vi "Cluster_Analysis.vi"(2 "Shift In":T1[](array[typedef])) -> (0 "Shift Out":T1[](array[typedef]))   [LabVIEW 2016]
uses:
  Controls/Shift_Cluster.ctl
  Controls/Inst_type.ctl
  Controls/XY_Plot_Cluster.ctl
  Globals/Meas_global.vi
  Globals/LDA_meas_global_1.vi
  Globals/LDA_meas_global_2.vi
  <vilib>/Analysis/NI_AALBase.lvlib
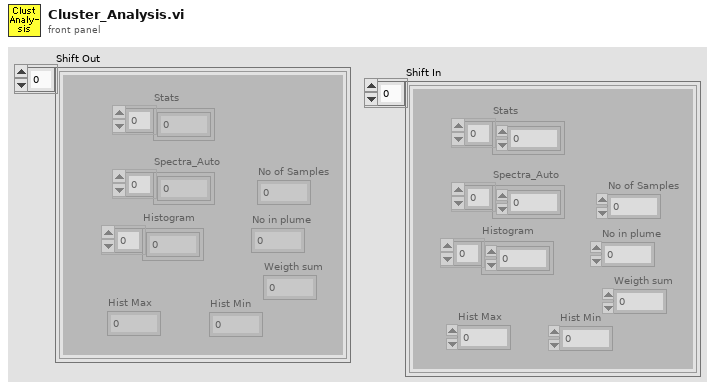
[diagram p1: front panel]
types:
  T1 = typedef "Shift_Cluster.ctl" = cluster{"Stats":dbl[], "Spectra_Auto":dbl[], "Histogram":dbl[], "Hist Max":dbl, "Hist Min":dbl, "No of Samples":i32, "No in plume":i32, "Weigth sum":dbl}
  T2 = typedef "Analysis_info_cluster.ctl" = cluster{"Colour":u32, "Inst type":T3, "Inst name":string, "Symbol":string, "Code name":string, "Extra Info":string, "Inst Array":T4, "Extra Titles":string[], "Extra Values":string[], "U":dbl, "u^2":dbl, "u^3":dbl, "u^4":dbl, "Skew_u":dbl, "Kurt_u":dbl, "Sd Error in Mean":dbl, "% u'/U":dbl, "X":dbl, "Y":dbl, "Z":dbl, "Timescale integral Estimate":dbl, "Sd Error in Variance":dbl, "Calib File":path, "Calib Constants":dbl[], "Output Position":bool, "Full Stats":bool, "Av Sampling Rate":dbl, "Av No of Samples":dbl, "Total Meas Time (s)":dbl, "ADAM Ch Name":string, "Max value":dbl, "Min value":dbl}
  T3 = typedef "Inst_type.ctl" = enum16{"Propeller anemometer", "Raw voltage", "Pressure Transducer", "Pitot-static tube", "Preston tube", "Hot wire", "Cross wire 1", "Cross wire 2", "Generic Linear", "Generic Polynomial", "Generic BackPoly", "Fast FID", "Thermocouple", "Cold wire", "Pulsed Wire", "LDA Vel", "LDA Tran time", "LDA Arr time", "Microphone"}
  T4 = typedef "Instrument_Array.ctl" = enum16{"PWA", "LDA", "Analogue"}
  T5 = typedef "Time_Trace_Cluster.ctl" = cluster{"Weighting":dbl[], "Time (s)":dbl[], "Voltage":dbl[], "Eng Values":dbl[]}
  T6 = typedef "XY_Plot_Cluster.ctl" = cluster{"First Name":string, "Second Name":string, "X axis name":string, "Y axis name":string, "X array":dbl[], "Y array":dbl[]}
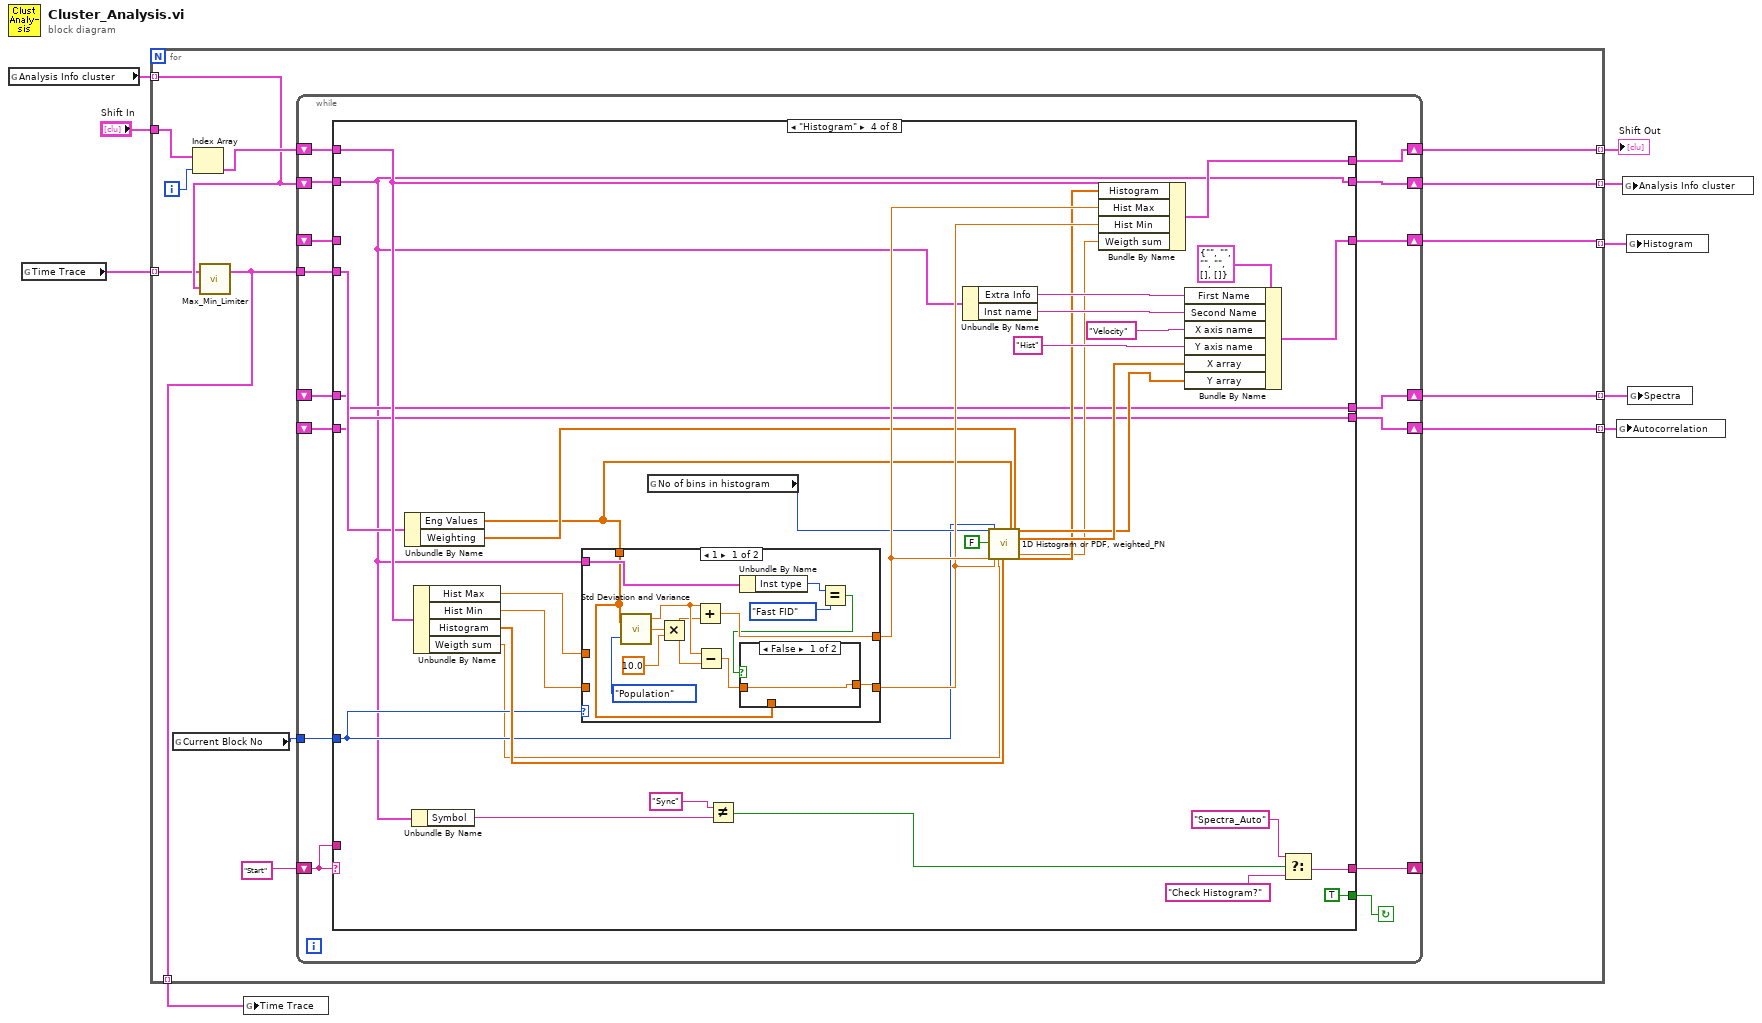
[diagram p0: block diagram]
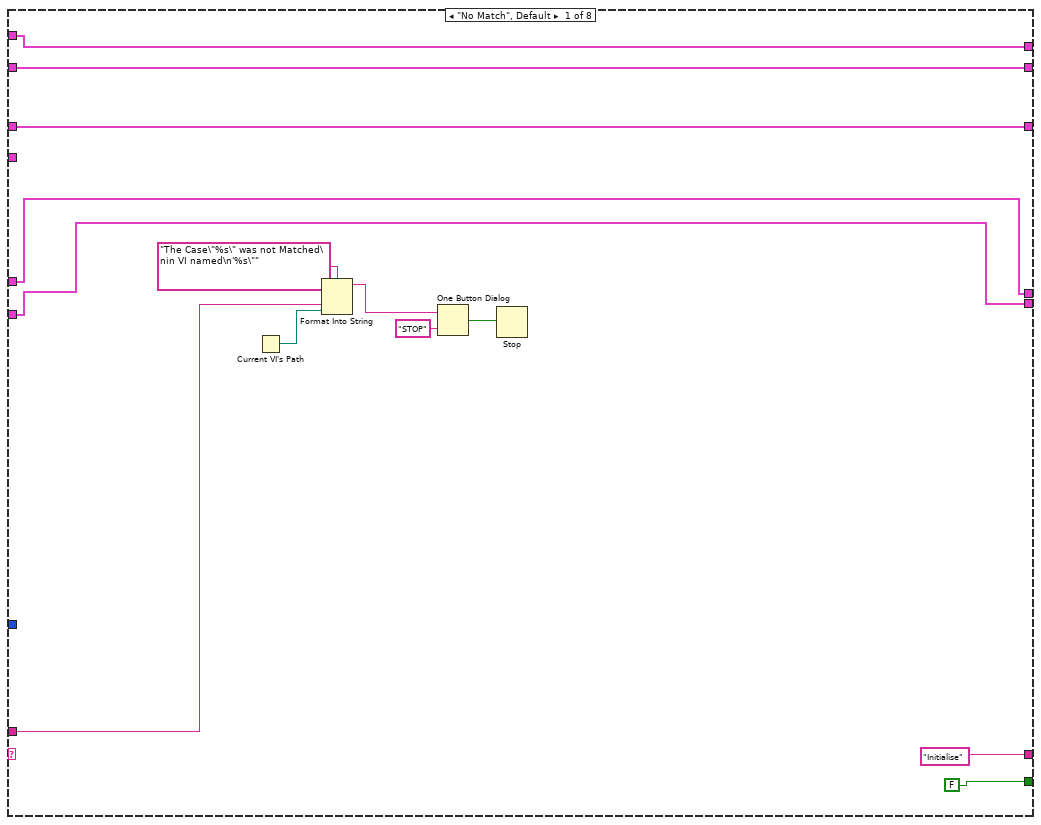
[diagram p2: hidden frame]
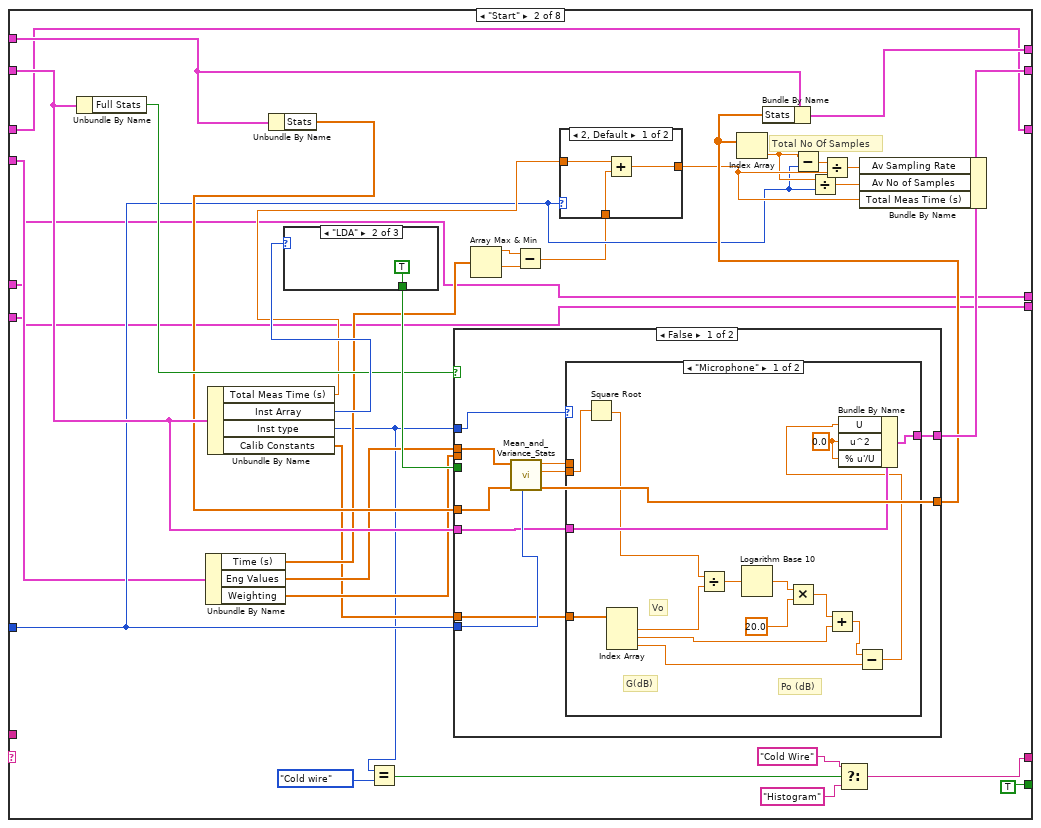
[diagram p3: hidden frame]
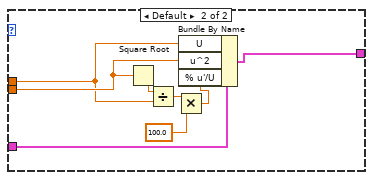
[diagram p5: hidden frame]
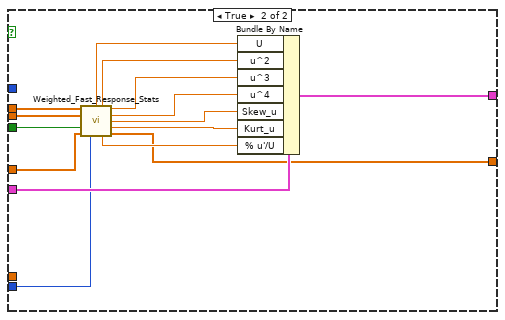
[diagram p6: hidden frame]
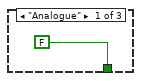
[diagram p7: hidden frame]
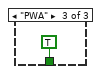
[diagram p8: hidden frame]
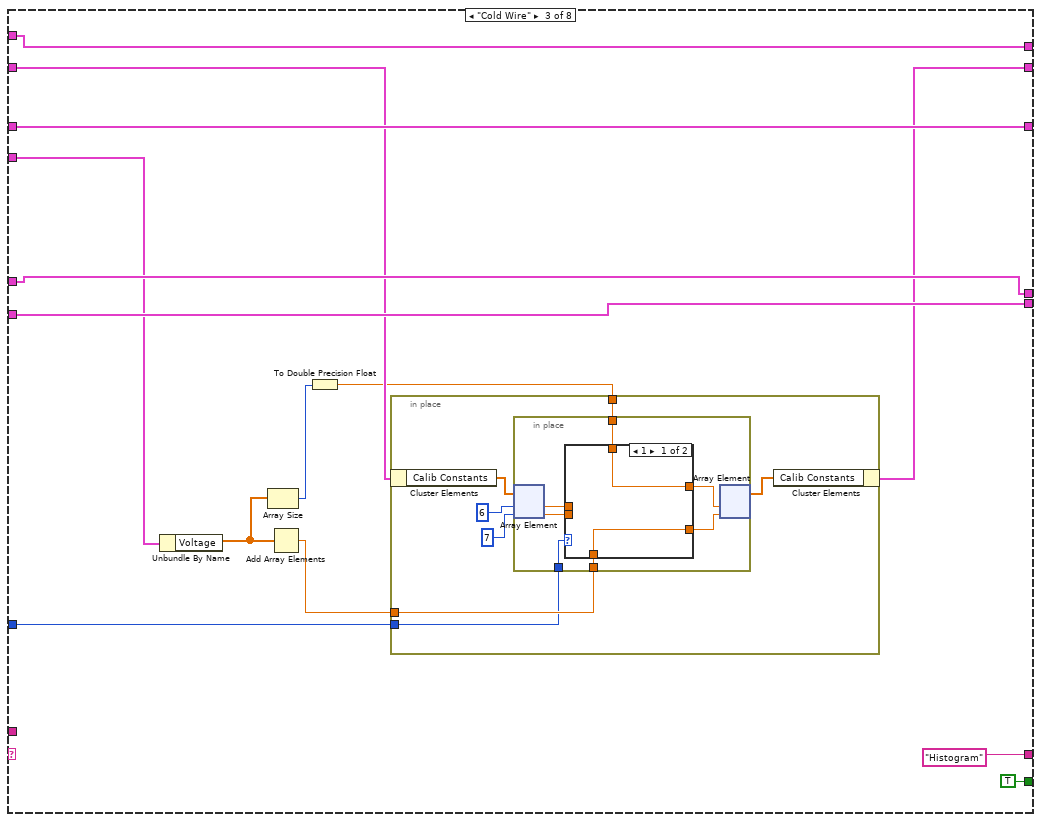
[diagram p9: hidden frame]
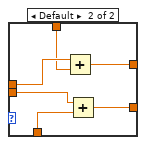
[diagram p10: hidden frame]
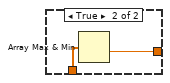
[diagram p11: hidden frame]
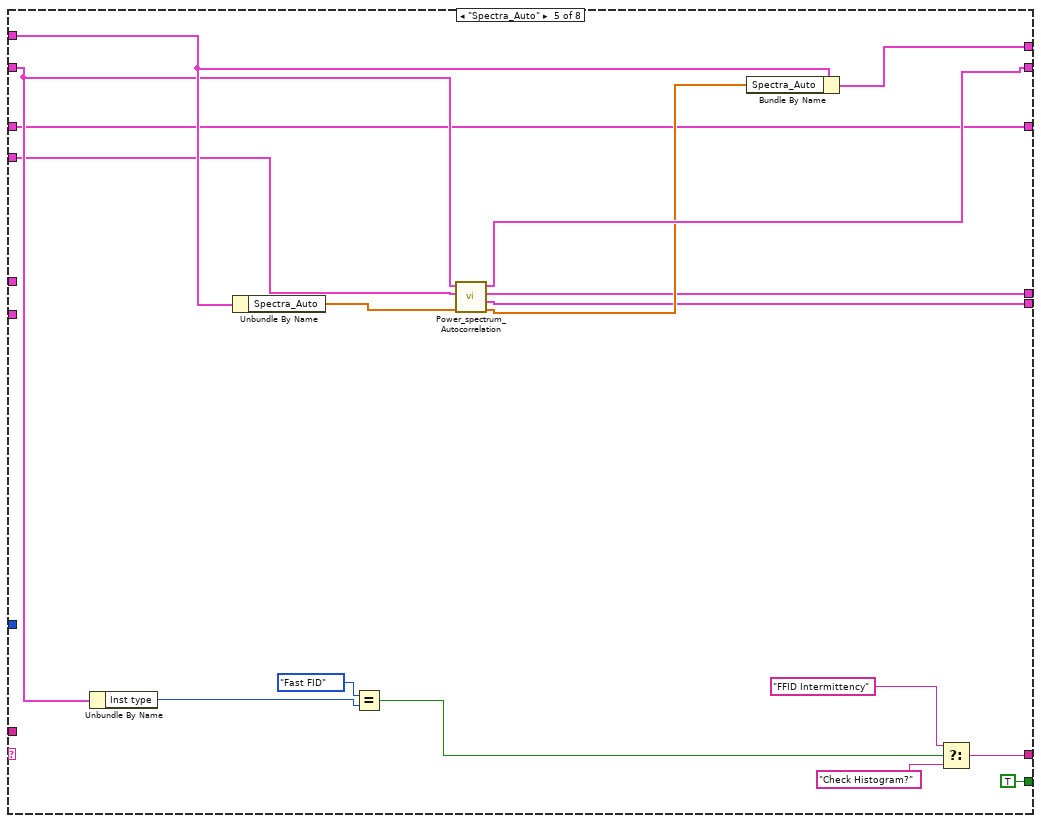
[diagram p13: hidden frame]
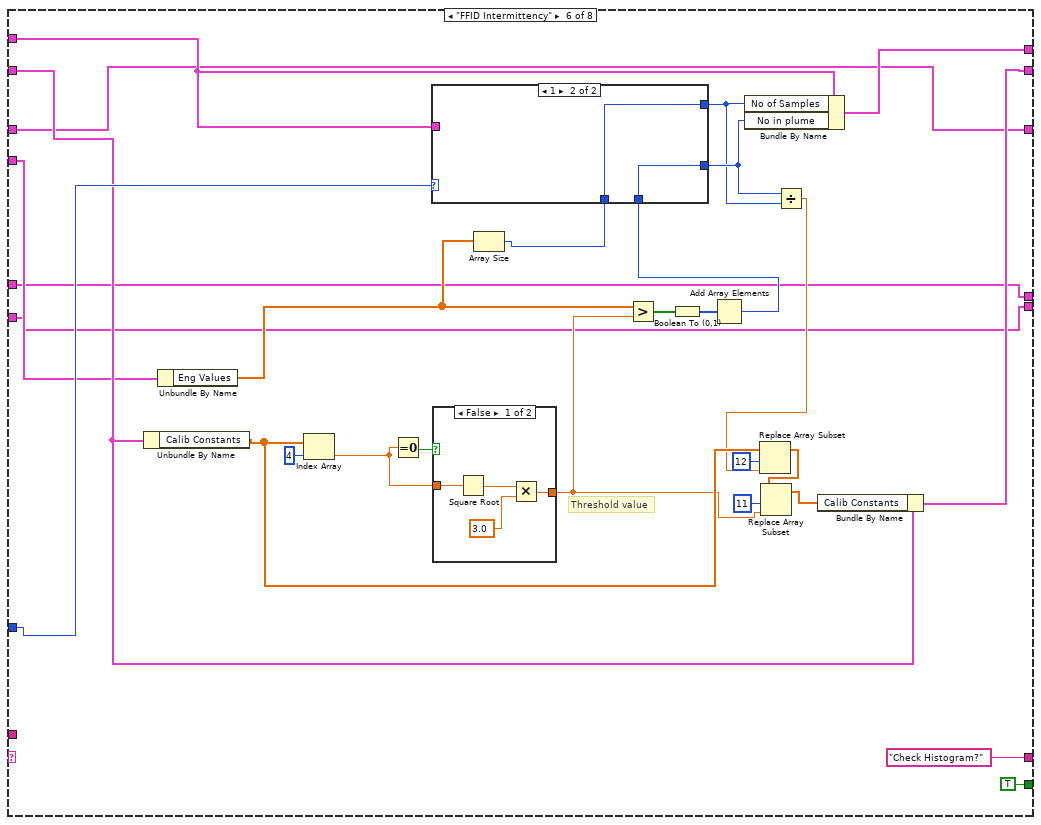
[diagram p14: hidden frame]
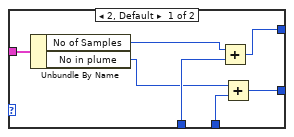
[diagram p15: hidden frame]
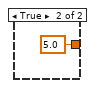
[diagram p16: hidden frame]
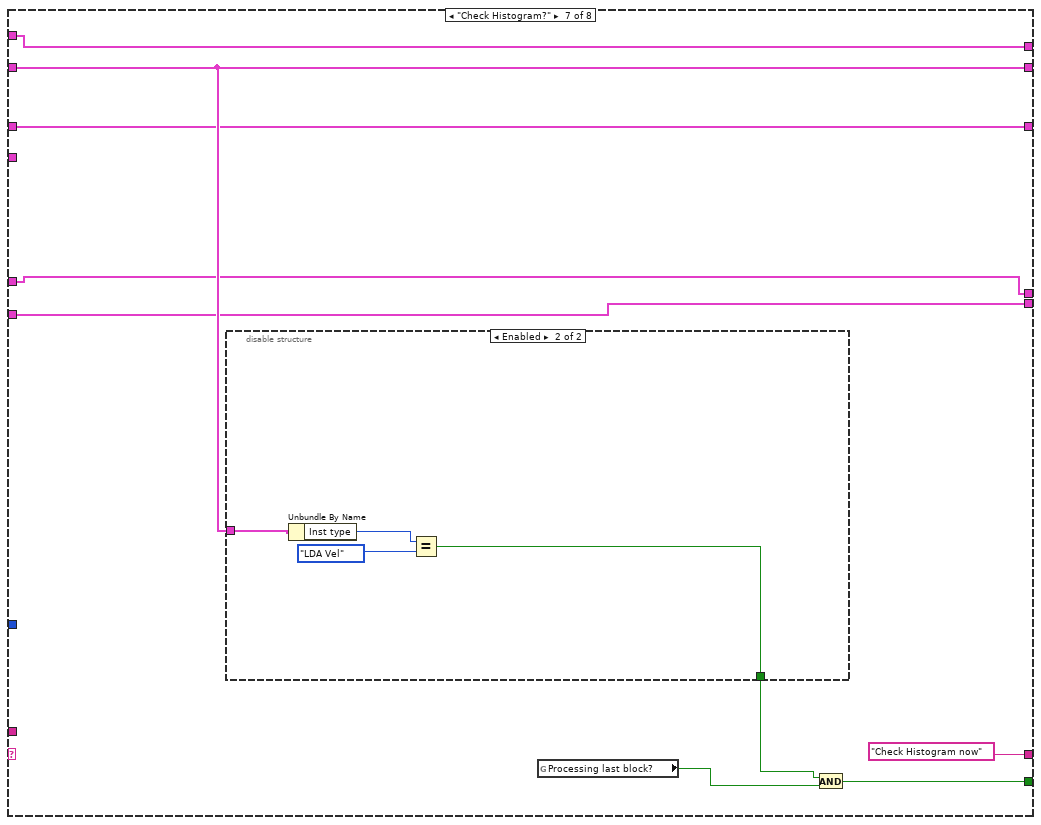
[diagram p17: hidden frame]
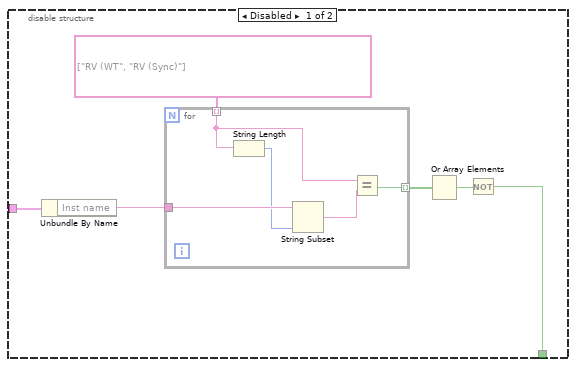
[diagram p18: hidden frame]
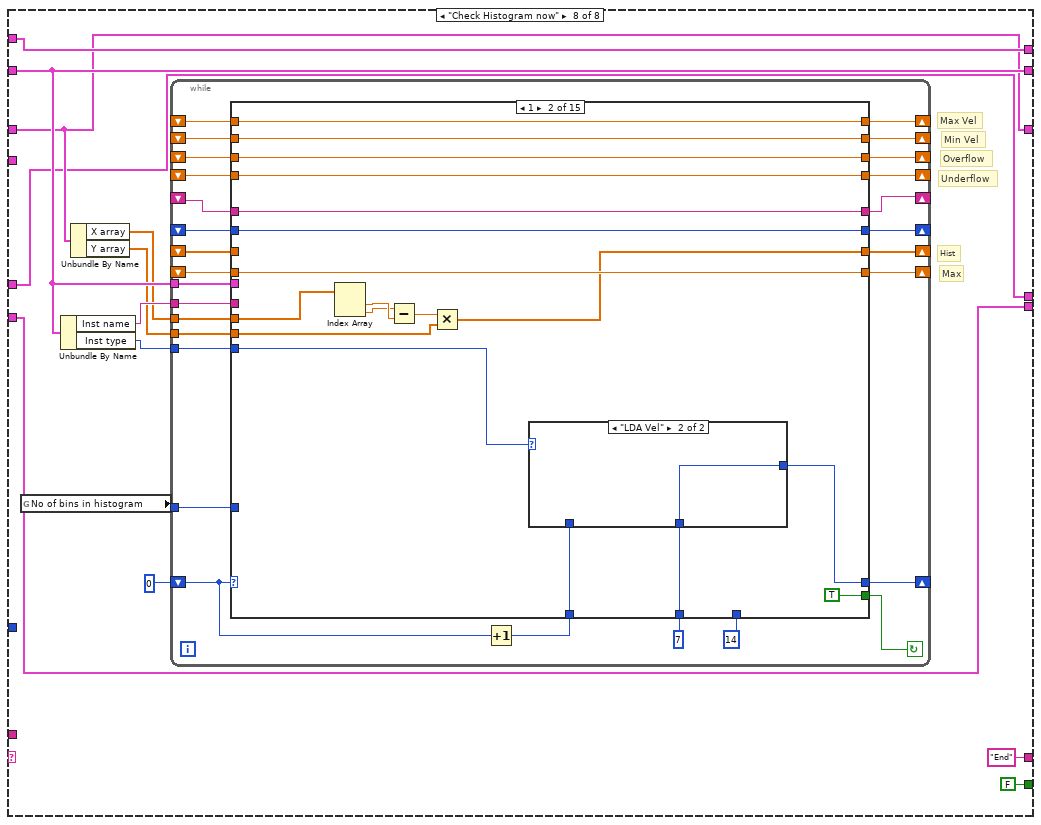
[diagram p19: hidden frame]
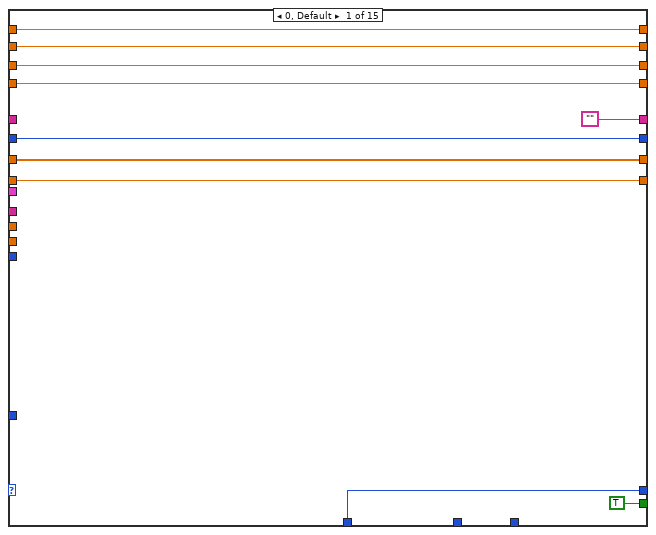
[diagram p20: hidden frame]
diagram:
  n1 = global read "Meas_global.vi" "Analysis Info cluster"() -> (w9:T2[])
  n2 = global read "Meas_global.vi" "Time Trace"() -> (w5:T5[])
  n3 = for {
    tunnel: "Shift In" -> [w20]
    tunnel: w9 -> [w12] mode=indexing
    tunnel: [w18] -> w7 mode=indexing
    tunnel: [w17] -> w6 mode=indexing
    tunnel: w5 -> [w11] mode=indexing
    tunnel: [w16] -> w4 mode=indexing
    tunnel: [w14] -> w2 mode=indexing
    tunnel: [w13] -> w3 mode=indexing
    tunnel: [w10] -> w1 mode=indexing
    i -> [w15]
    n4 = global read "Meas_global.vi" "Current Block No"() -> (w21:i32)
    n5 = Index Array(array=w20, index=w15) -> (element=w19:T1)
    n6 = call "Max_Min_Limiter.vi"("Analysis info"=w12, "Time Trace In"=w11) -> ("Time Trace Out"=w10:T5)  [unwired: 1 in]
    n7 = while {
      shift-left: "Start" -> [w35]
      shift-right: [w36] -> _
      shift-right: [w33] -> w17
      shift-left: w12 -> [w34]
      shift-right: [w31] -> w18
      shift-left: w19 -> [w32]
      tunnel: w21 -> [w30]
      tunnel: w10 -> [w29]
      shift-right: [w27] -> w16
      shift-left: _ -> [w28]
      shift-right: [w26] -> w14
      shift-left: _ -> [w24]
      shift-right: [w25] -> w13
      shift-left: _ -> [w23]
      stop <- w37 continue-if-true
      n8 = case shown="\"Histogram\"" w35 {
        tunnel: [FALSE TRUE TRUE ("Processing last block?") TRUE ("Processing last block?") TRUE ("Processing last block?") TRUE ("Full Stats") w292 FALSE ("Processing last block?")] -> w37
        tunnel: ["Initialise" w54 "Histogram" w200 w235 "Check Histogram?" "Check Histogram now" ("f") "End" ("f")] -> w36
        tunnel: w35 -> [w46 _ _ _ _ _ _ _]
        tunnel: w34 -> [w42 w82 w146 w177 w240 w260 w295 w317]
        tunnel: [w42 w74 w145 w177 w243 w259 w295 w317] -> w33
        tunnel: w32 -> [w41 w80 w154 w210 w245 w273 w296 w324]
        tunnel: [w41 w78 w154 w209 w244 w272 w296 w324] -> w31
        tunnel: w30 -> [_ w66 w142 w187 _ w265 _ _]
        tunnel: w29 -> [_ w65 w148 w184 w232 w250 _ _]
        tunnel: w28 -> [w40 w61 w153 _ w233 w248 w290 w316]
        tunnel: [w40 w61 w153 w181 w233 w248 w290 w316] -> w27
        tunnel: [w39 w59 w152 w179 w231 w247 w289 w313] -> w26
        tunnel: [w38 w60 w151 w178 w230 w246 w288 w312] -> w25
        tunnel: w24 -> [w39 w59 w152 w179 _ w247 w289 w313]
        tunnel: w23 -> [w38 w60 w151 w178 _ w246 w288 w312]
        frame "No Match", Default {
          n9 = Current VI's Path() -> (path=w45:path)
          n10 = Format Into String(format string="The Case\"%s\" was not Matched\nin VI named\n'%s\"" ("Format String"), w46, w45) -> (resulting string=w49:string)  [unwired: 2 in, 1 out]
          n11 = One Button Dialog(message=w49, button name ("OK")="STOP") -> (true=w47:bool)
          n12 = Stop(stop? (T)=w47) -> ()
        }
        frame "Start" {
          # "Total No Of Samples"
          n13 = Unbundle By Name(w82) -> ("Full Stats"=w81:bool)
          n14 = Unbundle By Name(w65) -> ("Time (s)"=w64:dbl[], "Eng Values"=w63:dbl[], "Weighting"=w62:dbl[])
          n15 = Unbundle By Name(w82) -> ("Total Meas Time (s)"=w73:dbl, "Inst Array"=w84:T4, "Inst type"=w52:T3, "Calib Constants"=w57:dbl[])
          n16 = Unbundle By Name(w80) -> ("Stats"=w79:dbl[])
          n17 = case shown="\"LDA\"" w84 {
            tunnel: [FALSE TRUE TRUE] -> w83
            frame "Analogue" {
            }
            frame "LDA" {
            }
            frame "PWA" {
            }
          }
          n18 = Equal?(x=w52, y=Inst_type."Cold wire" ("Inst type")) -> (x = y?=w51:bool)
          n19 = case shown="False" w81 {
            tunnel: w62 -> [_ w130]
            tunnel: w63 -> [w99 w129]
            tunnel: w83 -> [_ w128]
            tunnel: w82 -> [w97 w127]
            tunnel: w79 -> [w95 w126]
            tunnel: [w94 w125] -> w72
            tunnel: [w96 w124] -> w75
            tunnel: w66 -> [w98 w123]
            tunnel: w52 -> [w91 _]
            tunnel: w57 -> [w90 _]
            frame False {
              n20 = call "Mean_and_Variance_Stats.vi"("Block No"=w98, "Shift in"=w95, "U"=w99) -> ("Shift out"=w94:dbl[], "u^2"=w93:dbl, "U"=w92:dbl)  [unwired: 3 in]
              n21 = case shown="\"Microphone\"" w91 {
                tunnel: w97 -> [w114 w122]
                tunnel: [w113 w121] -> w96
                tunnel: w93 -> [w112 w120]
                tunnel: w92 -> [_ w118]
                tunnel: w90 -> [w102 _]
                frame "Microphone" {
                  w111 = 0.0 ("u^2")
                  # "Po (dB)"
                  # "G(dB)"
                  # "Vo"
                  n22 = Square Root(x=w112) -> (sqrt(x)=w101:dbl)
                  n23 = Index Array(array=w102) -> (element #1=w103:dbl, element #2=w108:dbl, element #3=w110:dbl)  [unwired: 3 in]
                  n24 = Divide(x=w101, y=w103) -> (x/y=w104:dbl)
                  n25 = Logarithm Base 10(1:w104) -> (0:w105:dbl)
                  n26 = Multiply(x=w105, y=20.0) -> (x*y=w107:dbl)
                  n27 = Add(x=w107, y=w108) -> (x+y=w109:dbl)
                  n28 = Subtract(x=w109, y=w110) -> (x-y=w100:dbl)
                  n29 = Bundle By Name(cluster=w114, "U"=w100, "u^2"=w111, "% u'/U"=w111) -> (w113:T2)
                }
                frame Default {
                  n30 = Square Root(x=w120) -> (sqrt(x)=w119:dbl)
                  n31 = Divide(x=w119, y=w118) -> (x/y=w117:dbl)
                  n32 = Multiply(x=w117, y=100.0) -> (x*y=w115:dbl)
                  n33 = Bundle By Name(cluster=w122, "U"=w118, "u^2"=w120, "% u'/U"=w115) -> (w121:T2)
                }
              }
            }
            frame True {
              n34 = call "Weighted_Fast_Response_Stats.vi"("U"=w129, "Weighting"=w130, "Use Weighting?"=w128, "Shift in"=w126, "Block No"=w123) -> ("U"=w131:dbl, "u^2"=w132:dbl, "u^3"=w133:dbl, "u^4"=w134:dbl, "Skew"=w135:dbl, "Kurt"=w136:dbl, "% u'/U"=w137:dbl, "Shift out"=w125:dbl[])  [unwired: 3 in]
              n35 = Bundle By Name(cluster=w127, "U"=w131, "u^2"=w132, "u^3"=w133, "u^4"=w134, "Skew_u"=w135, "Kurt_u"=w136, "% u'/U"=w137) -> (w124:T2)
            }
          }
          n36 = Array Max & Min(array=w64) -> (max value=w77:dbl, min value=w76:dbl)  [unwired: 2 out]
          n37 = Subtract(x=w77, y=w76) -> (x-y=w58:dbl)
          n38 = case shown="2, Default" w66 {
            tunnel: w58 -> [w88 w89]
            tunnel: w73 -> [w87 _]
            tunnel: [w86 w89] -> w70
            frame 2, Default {
              n39 = Add(x=w87, y=w88) -> (x+y=w86:dbl)
            }
            frame 1 {
            }
          }
          n40 = Index Array(array=w72) -> (element=w68:dbl)  [unwired: 1 in]
          n41 = Bundle By Name(cluster=w80, "Stats"=w72) -> (w78:T1)
          n42 = Subtract(x=w68, y=w66) -> (x-y=w67:dbl)
          n43 = Divide(x=w68, y=w66) -> (x/y=w69:dbl)
          n44 = Divide(x=w67, y=w70) -> (x/y=w71:dbl)
          n45 = Select(t="Cold Wire", s=w51, f="Histogram") -> (s? t:f=w54:string)
          n46 = Bundle By Name(cluster=w75, "Av Sampling Rate"=w71, "Av No of Samples"=w69, "Total Meas Time (s)"=w70) -> (w74:T2)
        }
        frame "Cold Wire" {
          n47 = Unbundle By Name(w148) -> ("Voltage"=w147:dbl[])
          n48 = Array Size(array=w147) -> (size(s)=w144:i32)
          n49 = Add Array Elements(numeric array=w147) -> (sum=w143:dbl)
          n50 = To Double Precision Float(number=w144) -> (double precision float=w141:dbl)
          n51 = in-place {
            in-place-border: w141 -> [w158]
            in-place-border: w143 -> [w157]
            in-place-border: w142 -> [w156]
            n52 = in-place-cluster #1(w146) -> ("Calib Constants"=w161:dbl[])
            n53 = in-place {
              in-place-border: w158 -> [w164]
              in-place-border: w157 -> [w163]
              in-place-border: w156 -> [w162]
              n54 = in-place-array #2(w161, 6, 7) -> (w168:dbl, w166:dbl)
              n55 = case shown="1" w162 {
                tunnel: w168 -> [_ w176]
                tunnel: [w170 w175] -> w167
                tunnel: w166 -> [_ w174]
                tunnel: [w169 w173] -> w165
                tunnel: w164 -> [w170 w172]
                tunnel: w163 -> [w169 w171]
                frame 1 {
                }
                frame Default {
                  n56 = Add(x=w176, y=w172) -> (x+y=w175:dbl)
                  n57 = Add(x=w174, y=w171) -> (x+y=w173:dbl)
                }
              }
              n58 = in-place-array #2(w167, w165) -> (w160:dbl[])  [unwired: 2 out]
            }
            n59 = in-place-cluster #1("Calib Constants"=w160) -> (w145:T2)
          }
        }
        frame "Histogram" {
          n60 = Unbundle By Name(w184) -> ("Eng Values"=w182:dbl[], "Weighting"=w183:dbl[])
          n61 = Unbundle By Name(w177) -> ("Symbol"=w197:string)
          n62 = Unbundle By Name(w210) -> ("Hist Max"=w208:dbl, "Hist Min"=w207:dbl, "Histogram"=w195:dbl[], "Weigth sum"=w186:dbl)
          n63 = case shown="1" w187 {
            tunnel: [w219 w228] -> w194
            tunnel: [w212 w227] -> w193
            tunnel: w182 -> [w213 _]
            tunnel: w208 -> [_ w228]
            tunnel: w207 -> [_ w227]
            tunnel: w177 -> [w217 _]
            frame 1 {
              n64 = call <vilib>:"Std Deviation and Variance.vi"("X"=w213, "Weighting (Sample)"=enum16{"Sample", "Population"}."Population") -> ("mean"=w223:dbl, "standard deviation"=w222:dbl)  [unwired: 1 out]
              n65 = Multiply(x=w222, y=10.0) -> (x*y=w220:dbl)
              n66 = Add(x=w223, y=w220) -> (x+y=w219:dbl)
              n67 = Subtract(x=w223, y=w220) -> (x-y=w211:dbl)
              n68 = Unbundle By Name(w217) -> ("Inst type"=w215:T3)
              n69 = Equal?(x=w215, y=Inst_type."Fast FID" ("Inst type")) -> (x = y?=w214:bool)
              n70 = case shown="False" w214 {
                tunnel: w213 -> [_ w226]
                tunnel: [w224 w225] -> w212
                tunnel: w211 -> [w224 _]
                frame False {
                }
                frame True {
                  n71 = Array Max & Min(array=w226) -> (min value=w225:dbl)  [unwired: 3 out]
                }
              }
            }
            frame 2, Default {
            }
          }
          n72 = global read "Meas_global.vi" "No of bins in histogram"() -> (w188:i32)
          n73 = Not Equal?(x="Sync", y=w197) -> (x != y?=w196:bool)
          n74 = Unbundle By Name(w177) -> ("Extra Info"=w204:string, "Inst name"=w203:string)
          n75 = call "1D Histogram or PDF, weighted_PN.vi"("Nbins"=w188, "Mean shift"=FALSE, "max"=w194, "Current block no."=w187, "min"=w193, "Shift SumW in"=w186, "Shift PDF in"=w195, "1D data"=w182, "Weights"=w183) -> ("1D histogram or PDF"=w191:dbl[], "bin centre vals."=w192:dbl[], "Shift SumW out"=w185:dbl, "Shift PDF out"=w190:dbl[])  [unwired: 14 in, 1 out]
          n76 = Bundle By Name(cluster=w210, "Histogram"=w190, "Hist Max"=w194, "Hist Min"=w193, "Weigth sum"=w185) -> (w209:T1)
          n77 = Bundle By Name(cluster=T6 {"First Name"="", "Second Name"="", "X axis name"="", "Y axis name"="", "X array"=[], "Y array"=[]} ("element"), "First Name"=w204, "Second Name"=w203, "X axis name"="Velocity", "Y axis name"="Hist", "X array"=w192, "Y array"=w191) -> (w181:T6)
          n78 = Select(t="Spectra_Auto", s=w196, f="Check Histogram?") -> (s? t:f=w200:string)
        }
        frame "Spectra_Auto" {
          n79 = Unbundle By Name(w240) -> ("Inst type"=w229:T3)
          n80 = Unbundle By Name(w245) -> ("Spectra_Auto"=w242:dbl[])
          n81 = Equal?(x=Inst_type."Fast FID" ("Inst type"), y=w229) -> (x = y?=w238:bool)
          n82 = call "Power_spectrum_Autocorrelation.vi"("Spectrum input array"=w242, "Time Trace"=w232, "Cluster in"=w240) -> ("Spectrum output array"=w241:dbl[], "Autocorrelation"=w230:T6, "Spectra"=w231:T6, "Cluster Out"=w243:T2)  [unwired: 2 in]
          n83 = Bundle By Name(cluster=w245, "Spectra_Auto"=w241) -> (w244:T1)
          n84 = Select(t="FFID Intermittency", s=w238, f="Check Histogram?") -> (s? t:f=w235:string)
        }
        frame "FFID Intermittency" {
          # "Threshold value"
          n85 = Unbundle By Name(w260) -> ("Calib Constants"=w258:dbl[])
          n86 = Unbundle By Name(w250) -> ("Eng Values"=w249:dbl[])
          n87 = Index Array(array=w258, index=4 ("Index")) -> (element=w268:dbl)
          n88 = Equal To 0?(x=w268) -> (x = 0?=w269:bool)
          n89 = case shown="False" w269 {
            tunnel: [w284 5.0] -> w253
            tunnel: w268 -> [w283 _]
            frame False {
              n90 = Square Root(x=w283) -> (sqrt(x)=w286:dbl)
              n91 = Multiply(x=w286, y=3.0) -> (x*y=w284:dbl)
            }
            frame True {
            }
          }
          n92 = Array Size(array=w249) -> (size(s)=w264:i32)
          n93 = Greater?(x=w249, y=w253) -> (0:w266:bool[])
          n94 = Boolean To (0,1)(Boolean=w266) -> (0, 1=w267:i16[])
          n95 = Add Array Elements(numeric array=w267) -> (sum=w263:i16)
          n96 = case shown="1" w265 {
            tunnel: w273 -> [w280 _]
            tunnel: w264 -> [w278 w281]
            tunnel: w263 -> [w277 w282]
            tunnel: [w276 w282] -> w262
            tunnel: [w275 w281] -> w261
            frame 2, Default {
              n97 = Unbundle By Name(w280) -> ("No of Samples"=w279:i32, "No in plume"=w274:i32)
              n98 = Add(x=w279, y=w278) -> (x+y=w275:i32)
              n99 = Add(x=w274, y=w277) -> (x+y=w276:i32)
            }
            frame 1 {
            }
          }
          n100 = Bundle By Name(cluster=w273, "No of Samples"=w261, "No in plume"=w262) -> (w272:T1)
          n101 = Divide(x=w262, y=w261) -> (x/y=w257:dbl)
          n102 = Replace Array Subset(array=w258, new element=w257, index=12) -> (w254:dbl[])
          n103 = Replace Array Subset(array=w254, new element=w253, index=11) -> (w252:dbl[])
          n104 = Bundle By Name(cluster=w260, "Calib Constants"=w252) -> (w259:T2)
        }
        frame "Check Histogram?" {
          n105 = disable-structure shown="Enabled" {
            disable-tunnel: w295 -> [w302 w311]
            disable-tunnel: [w297 w308] -> w291
            frame Disabled {
              n106 = Unbundle By Name(w302) -> ("Inst name"=w300:string)
              n107 = for {
                tunnel: string[] ["RV (WT", "RV (Sync)"] ("appended array") -> [w304] mode=indexing
                tunnel: w300 -> [w307]
                tunnel: [w303] -> w299 mode=indexing
                n108 = String Length(string=w304) -> (length=w306:i32)
                n109 = String Subset(string=w307, length (rest)=w306) -> (substring=w305:string)  [unwired: 1 in]
                n110 = Equal?(x=w304, y=w305) -> (x = y?=w303:bool)
              }
              n111 = Or Array Elements(Boolean array=w299) -> (logical OR=w298:bool)
              n112 = Not(x=w298) -> (.not. x?=w297:bool)
            }
            frame Enabled {
              n113 = Unbundle By Name(w311) -> ("Inst type"=w309:T3)
              n114 = Equal?(x=w309, y=Inst_type."LDA Vel" ("Inst type")) -> (x = y?=w308:bool)
            }
          }
          n115 = global read "Meas_global.vi" "Processing last block?"() -> (w293:bool)
          n116 = And(x=w291, y=w293) -> (x .and. y?=w292:bool)
        }
        frame "Check Histogram now" {
          # "Underflow"
          # "Overflow"
          # "Min Vel"
          # "Max Vel"
          # "Max"
          # "Hist"
          n117 = global read "Meas_global.vi" "No of bins in histogram"() -> (w321:i32)
          n118 = Unbundle By Name(w317) -> ("Inst name"=w318:string, "Inst type"=w319:T3)
          n119 = Unbundle By Name(w316) -> ("X array"=w315:dbl[], "Y array"=w314:dbl[])
          n120 = while {
            tunnel: w321 -> [w340]
            shift-left: _ -> [w341]
            shift-right: [w343] -> _
            shift-left: _ -> [w342]
            shift-right: [w344] -> _
            shift-left: _ -> [w345]
            shift-right: [w346] -> _
            shift-left: _ -> [w347]
            shift-right: [w348] -> _
            shift-left: 0 -> [w351]
            shift-right: [w349] -> _
            shift-right: [w337] -> _
            shift-left: _ -> [w335]
            shift-right: [w336] -> _
            shift-left: _ -> [w334]
            shift-right: [w333] -> _
            shift-left: _ -> [w330]
            shift-right: [w332] -> _
            shift-left: _ -> [w331]
            tunnel: w319 -> [w329]
            tunnel: w315 -> [w328]
            tunnel: w314 -> [w327]
            tunnel: w318 -> [w326]
            tunnel: w317 -> [w325]
            stop <- w352 continue-if-true
            n121 = Increment(x=w351) -> (x+1=w350:i32)
            n122 = case shown="1" w351 {
              tunnel: [TRUE TRUE TRUE TRUE TRUE TRUE TRUE TRUE TRUE TRUE TRUE TRUE TRUE TRUE FALSE] -> w352
              tunnel: w350 -> [w362 w376 w390 w435 w466 w481 _ w526 w551 w586 w611 w632 w639 w660 w662]
              tunnel: [w362 w377 w388 w437 w466 w489 w515 w526 w551 w586 w613 w632 w641 w660 w662] -> w349
              tunnel: [w357 w379 w403 w423 w458 w472 w510 w528 w558 w593 w614 w628 w642 w656 w664] -> w348
              tunnel: w347 -> [w357 w379 w403 _ w458 _ w510 w528 w558 w593 w614 w628 w642 w656 w664]
              tunnel: ["" w378 w402 w436 w464 w488 w517 w530 w559 w594 w617 w630 w645 w658 w665] -> w346
              tunnel: w345 -> [_ w378 w402 w436 w465 w488 w518 w530 w559 w594 w617 w631 w645 w659 w665]
              tunnel: [w360 w363 w400 w428 w462 w478 w516 w529 w554 w589 w616 w629 w644 w657 w673] -> w344
              tunnel: [w359 w370 w401 w426 w461 w476 w512 w527 w552 w587 w615 w624 w643 w652 w672] -> w343
              tunnel: w342 -> [w360 _ w400 w428 w462 w478 w516 w529 w554 w589 w616 w629 w644 w657 w673]
              tunnel: w341 -> [w359 w370 w401 _ w461 _ w512 _ w552 w587 w615 w624 w643 w652 w672]
              tunnel: w340 -> [_ _ _ w429 _ w485 _ _ w540 w574 _ _ _ _ _]
              tunnel: 7 -> [_ w375 _ _ _ _ _ _ _ _ _ _ _ _ _]
              tunnel: 14 ("y") -> [_ _ w389 _ _ w480 w515 _ _ _ _ _ _ _ _]
              tunnel: [w356 w374 w386 w422 w456 w471 w508 w524 w546 w582 w609 w620 w637 w651 w671] -> w337
              tunnel: [w355 w373 w385 w421 w455 w470 w507 w523 w547 w581 w608 w623 w636 w648 w670] -> w336
              tunnel: w335 -> [w356 w374 w386 w422 w456 w471 w508 _ w546 w582 w609 w620 w637 w651 w671]
              tunnel: w334 -> [w355 w373 w385 w421 w455 w470 w507 _ w547 w581 w608 w623 w636 w648 w670]
              tunnel: [w353 w371 w383 w419 w453 w468 w505 w521 w545 w580 w606 w621 w635 w650 w668] -> w333
              tunnel: [w354 w372 w384 w420 w454 w469 w506 w522 w544 w579 w607 w622 w634 w649 w669] -> w332
              tunnel: w331 -> [w354 w372 w384 w420 w454 w469 w506 w522 w544 _ w607 w622 w634 w649 w669]
              tunnel: w330 -> [w353 w371 w383 w419 w453 w468 w505 w521 _ w580 w606 w621 w635 w650 w668]
              tunnel: w329 -> [_ w369 _ _ _ _ _ _ _ _ _ _ _ _ _]
              tunnel: w328 -> [_ w366 _ _ w451 _ w503 _ w536 w571 _ _ _ _ _]
              tunnel: w327 -> [_ w364 _ _ _ _ _ _ _ _ _ _ _ _ _]
              tunnel: w326 -> [_ _ _ _ w452 _ w504 _ _ _ _ w619 _ w647 _]
              tunnel: w325 -> [_ _ _ _ _ _ _ w520 _ _ _ _ _ _ _]
              frame 0, Default {
              }
              frame 1 {
                n123 = Index Array(array=w366) -> (element #1=w368:dbl, element #2=w367:dbl)  [unwired: 2 in]
                n124 = Subtract(x=w367, y=w368) -> (x-y=w365:dbl)
                n125 = Multiply(x=w365, y=w364) -> (x*y=w363:dbl[])
                n126 = case shown="\"LDA Vel\"" w369 {
                  tunnel: [w381 w382] -> w377
                  tunnel: w376 -> [w381 _]
                  tunnel: w375 -> [_ w382]
                  frame "Propeller anemometer", Default {
                  }
                  frame "LDA Vel" {
                  }
                }
              }
              frame 2 {
                n127 = for {
                  tunnel: w400 -> [w412] mode=indexing
                  shift-right: [w405] -> _
                  shift-left: FALSE -> [w411]
                  shift-right: [w408] -> w394
                  shift-left: 0 -> [w409]
                  shift-right: [w406] -> w396
                  shift-left: 0 -> [w407]
                  n128 = Greater Than 0?(x=w412) -> (x > 0?=w405:bool)
                  n129 = Compound Arithmetic op=AND(w405, invert w411) -> (w410:bool)
                  n130 = case shown="True" w405 {
                    tunnel: w407 -> [w413 w415]
                    tunnel: [w413 w414] -> w406
                    frame False {
                    }
                    frame True {
                      n131 = Increment(x=w415) -> (x+1=w414:i32)
                    }
                  }
                  n132 = case shown="True" w410 {
                    tunnel: w409 -> [w416 w418]
                    tunnel: [w416 w417] -> w408
                    frame False {
                    }
                    frame True {
                      n133 = Increment(x=w418) -> (x+1=w417:i32)
                    }
                  }
                }
                n134 = Equal?(x=w394, y=1) -> (x = y?=w391:bool)
                n135 = Greater?(x=w396, y=10) -> (0:w392:bool)
                n136 = And(x=w392, y=w391) -> (x .and. y?=w387:bool)
                n137 = Select(t=w390, s=w387, f=w389) -> (s? t:f=w388:i32)
              }
              frame 3 {
                # "Clipping?"
                n138 = Increment(x=w429) -> (x+1=w442:i32)
                n139 = while {
                  tunnel: [w443] -> w426
                  tunnel: w428 -> [w450]
                  shift-left: 0.0 -> [w443]
                  shift-right: [w448] -> w439
                  shift-left: w442 -> [w449]
                  shift-right: [w447] -> w425
                  stop <- w444 continue-if-true
                  n140 = Decrement(x=w449) -> (x-1=w447:i32)
                  n141 = Index Array(array=w450, index=w449) -> (element=w448:dbl)
                  n142 = Equal To 0?(x=w443) -> (x = 0?=w445:bool)
                  n143 = Greater Than 0?(x=w447) -> (x > 0?=w446:bool)
                  n144 = And(x=w446, y=w445) -> (x .and. y?=w444:bool)
                }
                n145 = Greater?(x=w426, y=0.04) -> (0:w431:bool)
                n146 = Multiply(x=w426, y=0.7) -> (x*y=w440:dbl)
                n147 = Add(x=w425, y=2) -> (x+y=w423:i32)
                n148 = Increment(x=w435) -> (x+1=w434:i32)
                n149 = Greater?(x=w440, y=w439) -> (0:w432:bool)
                n150 = And(x=w431, y=w432) -> (x .and. y?=w430:bool)
                n151 = Select(t=w435, s=w430, f=w434) -> (s? t:f=w437:i32)
              }
              frame 4 {
                n152 = Index Array(array=w451, index=w458) -> (element=w457:dbl)
                n153 = Multiply(x=w461, y=100.0) -> (x*y=w459:dbl)
                n154 = Format Into String(format string="Histogram of %s may indicate Clipping at Upper limit of %.2f by %.0f%%.\\n" ("Format String"), initial string=w465, w452, w457, w459) -> (resulting string=w464:string)  [unwired: 1 in, 1 out]
              }
              frame 5 {
                # "Clipping?"
                n155 = Array Max & Min(array=w478) -> (max value=w477:dbl)  [unwired: 3 out]
                n156 = while {
                  tunnel: w485 -> [w495]
                  tunnel: [w497] -> w476
                  tunnel: w478 -> [w502]
                  shift-left: 0.0 -> [w497]
                  shift-right: [w500] -> w491
                  shift-left: 0 -> [w501]
                  shift-right: [w496] -> w474
                  stop <- w498 continue-if-true
                  n157 = Increment(x=w501) -> (x+1=w496:i32)
                  n158 = Index Array(array=w502, index=w501) -> (element=w500:dbl)
                  n159 = Less?(x=w496, y=w495) -> (x < y?=w494:bool)
                  n160 = Equal To 0?(x=w497) -> (x = 0?=w499:bool)
                  n161 = And(x=w494, y=w499) -> (x .and. y?=w498:bool)
                }
                n162 = Not Equal?(x=w476, y=w477) -> (x != y?=w475:bool)
                n163 = Greater?(x=w476, y=0.04) -> (0:w483:bool)
                n164 = Multiply(x=w476, y=0.45) -> (x*y=w492:dbl)
                n165 = Subtract(x=w474, y=2) -> (x-y=w472:i32)
                n166 = Greater?(x=w492, y=w491) -> (0:w484:bool)
                n167 = Compound Arithmetic op=AND(w475, w483, w484) -> (w482:bool)
                n168 = Select(t=w481, s=w482, f=w480) -> (s? t:f=w489:i32)
              }
              frame 6 {
                n169 = Index Array(array=w503, index=w510) -> (element=w509:dbl)
                n170 = Multiply(x=w512, y=100.0) -> (x*y=w511:dbl)
                n171 = Format Into String(format string="Histogram of %s may indicate Clipping at Lower limit of %.2f by %.0f%%.\\n" ("Format String"), initial string=w518, w504, w509, w511) -> (resulting string=w517:string)  [unwired: 1 in, 1 out]
              }
              frame 7 {
                n172 = Unbundle By Name(w520) -> ("Code name"=w525:string)
                n173 = case shown="\"1LDA:U\", Default" w525 {
                  tunnel: [w533 w535] -> w524
                  tunnel: [w532 w534] -> w523
                  frame "1LDA:U", Default {
                    n174 = global read "LDA_meas_global_1.vi" "Max Vel BSA1"() -> (w533:dbl)
                    n175 = global read "LDA_meas_global_1.vi" "Min Vel BSA1"() -> (w532:dbl)
                  }
                  frame "2LDA:U" {
                    n176 = global read "LDA_meas_global_2.vi" "Max Vel BSA2"() -> (w535:dbl)
                    n177 = global read "LDA_meas_global_2.vi" "Min Vel BSA2"() -> (w534:dbl)
                  }
                }
                n178 = Add Array Elements(numeric array=w529) -> (sum=w527:dbl)
              }
              frame 8 {
                n179 = Divide(x=w540, y=2) -> (x/y=w538:dbl)
                n180 = Array Max & Min(array=w536) -> (max value=w543:dbl, min value=w542:dbl)  [unwired: 2 out]
                n181 = Subtract(x=w543, y=w542) -> (x-y=w541:dbl)
                n182 = Divide(x=w541, y=w538) -> (x/y=w537:dbl)
                n183 = Subtract(x=w546, y=w537) -> (x-y=w557:dbl)
                n184 = for {
                  tunnel: w557 -> [w564]
                  shift-right: [w562] -> w553
                  shift-left: 0.0 -> [w565]
                  tunnel: w554 -> [w566] mode=indexing
                  tunnel: w536 -> [w561] mode=indexing
                  n185 = Greater?(x=w561, y=w564) -> (0:w563:bool)
                  n186 = case shown="False" w563 {
                    tunnel: w566 -> [_ w569]
                    tunnel: w565 -> [w567 w570]
                    tunnel: [w567 w568] -> w562
                    frame False {
                    }
                    frame True {
                      n187 = Add(x=w570, y=w569) -> (x+y=w568:dbl)
                    }
                  }
                }
                n188 = Divide(x=w553, y=w552) -> (x/y=w549:dbl)
                n189 = Greater?(x=w549, y=0.025) -> (0:w550:bool)
                n190 = Select(t=w549, s=w550, f=0.0) -> (s? t:f=w545:dbl)
              }
              frame 9 {
                n191 = Divide(x=w574, y=2) -> (x/y=w573:dbl)
                n192 = Array Max & Min(array=w571) -> (max value=w578:dbl, min value=w577:dbl)  [unwired: 2 out]
                n193 = Subtract(x=w578, y=w577) -> (x-y=w576:dbl)
                n194 = Divide(x=w576, y=w573) -> (x/y=w572:dbl)
                n195 = Add(x=w581, y=w572) -> (x+y=w592:dbl)
                n196 = for {
                  tunnel: w592 -> [w599]
                  shift-right: [w597] -> w588
                  shift-left: 0.0 -> [w600]
                  tunnel: w589 -> [w601] mode=indexing
                  tunnel: w571 -> [w596] mode=indexing
                  n197 = Less?(x=w596, y=w599) -> (x < y?=w598:bool)
                  n198 = case shown="True" w598 {
                    tunnel: w601 -> [_ w604]
                    tunnel: w600 -> [w602 w605]
                    tunnel: [w602 w603] -> w597
                    frame False {
                    }
                    frame True {
                      n199 = Add(x=w605, y=w604) -> (x+y=w603:dbl)
                    }
                  }
                }
                n200 = Divide(x=w588, y=w587) -> (x/y=w584:dbl)
                n201 = Greater?(x=w584, y=0.025) -> (0:w585:bool)
                n202 = Select(t=w584, s=w585, f=0.0) -> (s? t:f=w579:dbl)
              }
              frame 10 {
                n203 = Equal To 0?(x=w606) -> (x = 0?=w612:bool)
                n204 = Increment(x=w611) -> (x+1=w610:i32)
                n205 = Select(t=w610, s=w612, f=w611) -> (s? t:f=w613:i32)
              }
              frame 11 {
                n206 = Multiply(x=w621, y=100.0) -> (x*y=w625:dbl)
                n207 = Format Into String(format string="%.1f %% of the %s samples are too close to the upper velocity limit of %.2f m/s.\n" ("Format String"), initial string=w631, w625, w619, w620) -> (resulting string=w630:string)  [unwired: 1 in, 1 out]
              }
              frame 12 {
                n208 = Equal To 0?(x=w634) -> (x = 0?=w640:bool)
                n209 = Increment(x=w639) -> (x+1=w638:i32)
                n210 = Select(t=w638, s=w640, f=w639) -> (s? t:f=w641:i32)
              }
              frame 13 {
                n211 = Multiply(x=w649, y=100.0) -> (x*y=w653:dbl)
                n212 = Format Into String(format string="%.1f %% of the %s samples are too close to the lower velocity limit of %.2f m/s.\n" ("Format String"), initial string=w659, w653, w647, w648) -> (resulting string=w658:string)  [unwired: 1 in, 1 out]
              }
              frame 14 {
                n213 = global read "Meas_global.vi" "Over/Under string"() -> (w667:string)
                n214 = Concatenate Strings(w667, w665) -> (w666:string)
                n215 = global write "Meas_global.vi" "Over/Under string"(w666) -> ()
              }
            }
          }
        }
      }
    }
  }
  "Shift Out" <- w7
  n216 = global write "Meas_global.vi" "Time Trace"(w1) -> ()
  n217 = global write "Meas_global.vi" "Autocorrelation"(w3) -> ()
  n218 = global write "Meas_global.vi" "Analysis Info cluster"(w6) -> ()
  n219 = global write "Meas_global.vi" "Histogram"(w4) -> ()
  n220 = global write "Meas_global.vi" "Spectra"(w2) -> ()
